vi "GoHome.vi"(8 "error in (no error)":errorcluster, 11 "Controlador in":refnum<class "Controlador.lvclass">) -> (0 "error out":errorcluster, 2 "String":string, 3 "Controlador out":refnum<class "Controlador.lvclass">)   [LabVIEW 2011]
uses:
  Controlador.lvclass
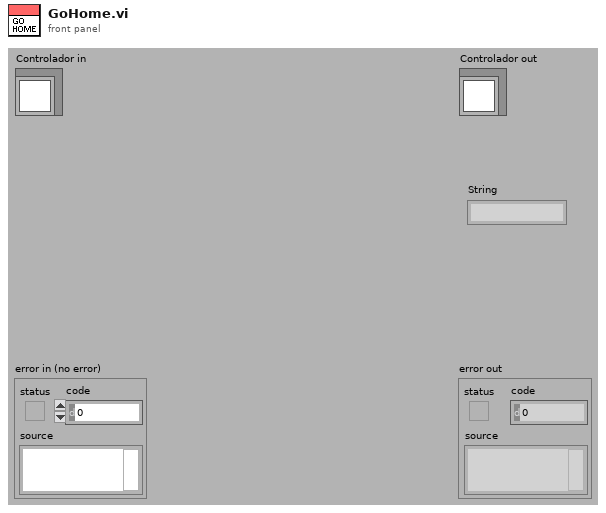
[diagram p1: front panel]
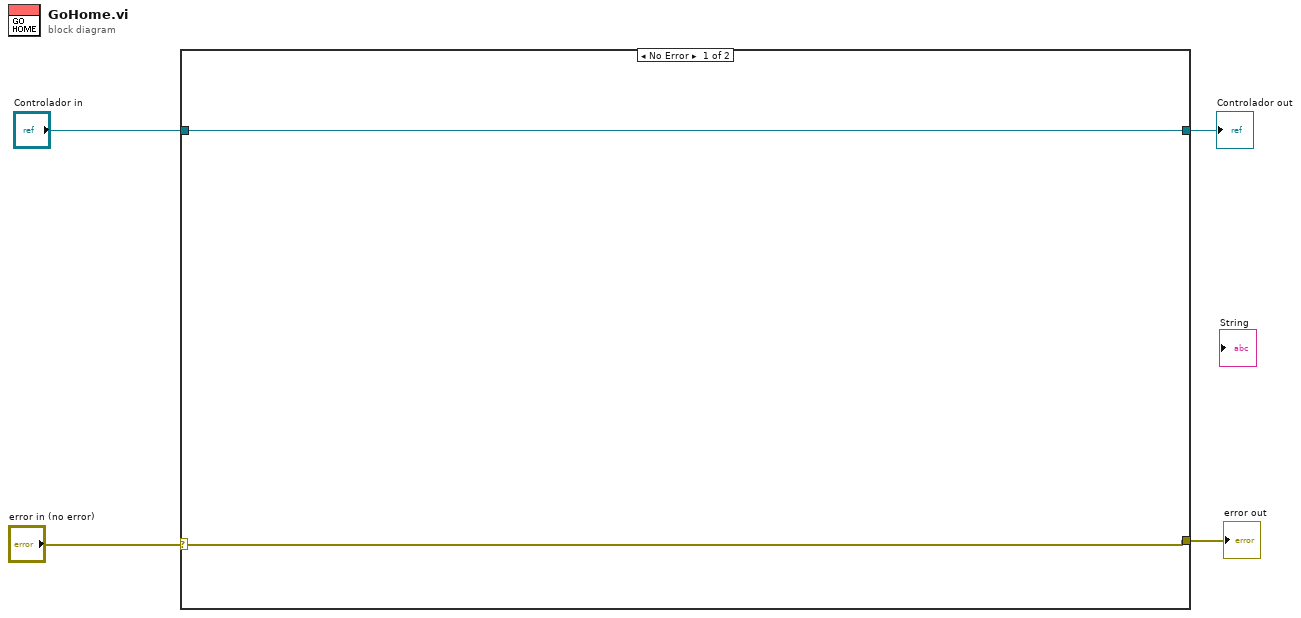
[diagram p0: block diagram]
diagram:
  n1 = case shown="No Error" "error in (no error)" {
    selector: "error in (no error)" -> [w5 w7]
    tunnel: [w5 w7] -> w3
    tunnel: "Controlador in" -> [w6 w8]
    tunnel: [w6 w8] -> w4
    frame No Error {
    }
    frame Error {
    }
  }
  "error out" <- w3
  "Controlador out" <- w4
